vi "Do.vi"(8 "error in (no error)":errorcluster, 10 "Actor in":refnum<class "Actor.lvclass">, 11 "Send Get Hardware Info Message":refnum<class "Send Get Hardware Info Message.lvclass">) -> (0 "error out":errorcluster, 2 "Actor out":refnum<class "Actor.lvclass">)   [LabVIEW 2017, in "Measurement UI.lvlib" / "Send Get Hardware Info Message.lvclass"]
uses:
  Send Get Hardware Info Message.lvclass
  <vilib>/ActorFramework/Actor/Actor.lvclass
  Measurement UI.lvclass
  C:/Program Files (x86)/National Instruments/LabVIEW 2017/vi.lib/ActorFramework/Actor/Actor.lvclass
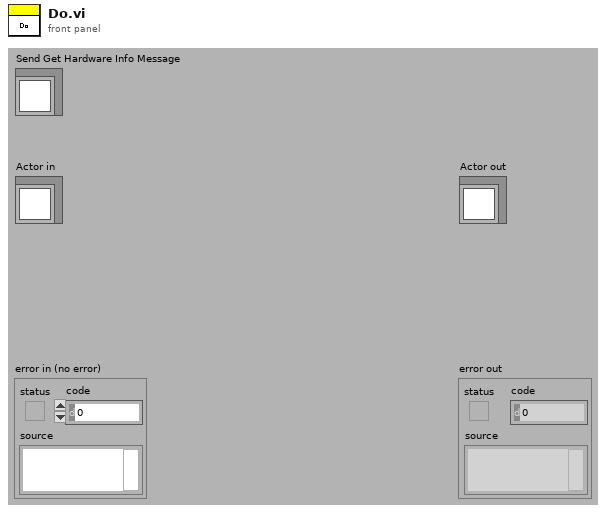
[diagram p1: front panel]
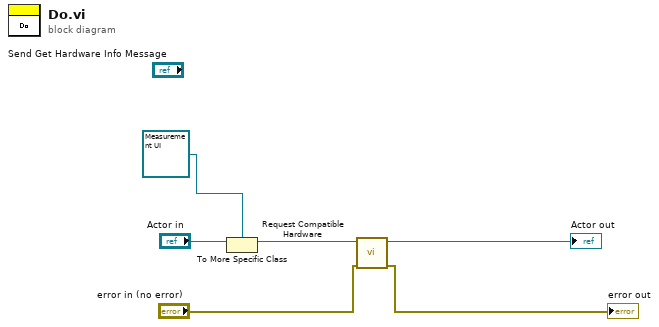
[diagram p0: block diagram]
diagram:
  n1 = To More Specific Class(target class=refnum<class "Measurement UI.lvclass"> refnum ("UI.lvclass"), reference="Actor in") -> (specific class reference=w4:refnum<class "Measurement UI.lvclass">)  [unwired: 1 in, 1 out]
  n2 = call-dynamic "Request Compatible Hardware.vi"("error in (no error)"="error in (no error)", "Msmt UI in"=w4) -> ("error out"=→"error out":errorcluster, "Msmt UI out"=→"Actor out":refnum<class "Measurement UI.lvclass">)  [unwired: 8 in]
